vi "Modbusd cmd to db.vi"(0 "reference in":refnum<class "Device.lvclass">, 5 "Data Read":T1, 11 "error in (no error)":errorcluster) -> (4 "reference out":refnum<class "Device.lvclass">, 15 "error out":errorcluster)   [LabVIEW 2019, in "Device.lvclass"]
uses:
  Device.lvclass
  C:/Users/ANENKOV_V1/Desktop/src/Proccess_class/Proccess.lvclass
  Modbus_class/ReadData.ctl
  Proccess_class/Proccess.lvclass/Proccess.ctl
  Logger_class/EventData.ctl
  TypeDef/AlarmType.ctl
  Logger_class/Logger.lvclass
  Proccess_class/Proccess.lvclass
  Modbus_class/ModbusSp.lvclass
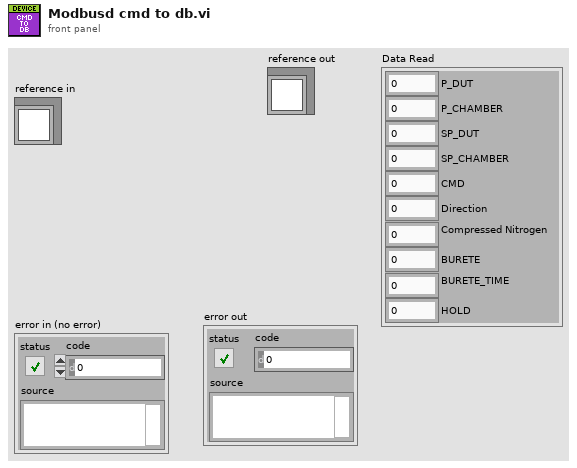
[diagram p1: front panel]
types:
  T1 = typedef "ModbusSp.lvclass/ReadData.ctl" = cluster{"P_DUT":sgl, "P_CHAMBER":sgl, "SP_DUT":sgl, "SP_CHAMBER":sgl, "CMD":u16, "Direction":u16, "Compressed Nitrogen":u16, "BURETE":u16, "BURETE_TIME":u16, "HOLD":u16}
  T2 = typedef "CMD REG.ctl" = cluster{"EXECUTE_SP":bool, "ALARM_PRESS_DOWN_DUT":bool, "ALARM_PRESS_DOWN_CHAMBER":bool, "ALARM_PRESS_DOWN_DUT_CHAMBER":bool, "FILING_DUT":bool, "FILING_CHAMBER":bool, "BLOCK":bool, "PUMP_STATION_OFF":bool, "Leak start":bool, "Leak stop":bool, "Drain":bool}
  T3 = typedef "EventData.ctl" = cluster{"obj_tag":string, "event_tag":string, "Description":string, "ALARM TYPE":T4, "Value DBL":dbl, "Value INT":i32, "Value STR":string, "Time Stamp":timestamp}
  T4 = typedef "AlarmType.ctl" = enum16{"Normal", "Warning", "Alarm"}
  T5 = typedef "Proccess.lvclass/TAGs.ctl" = cluster{"TAG":string, "PTAG":string, "DESC":string}
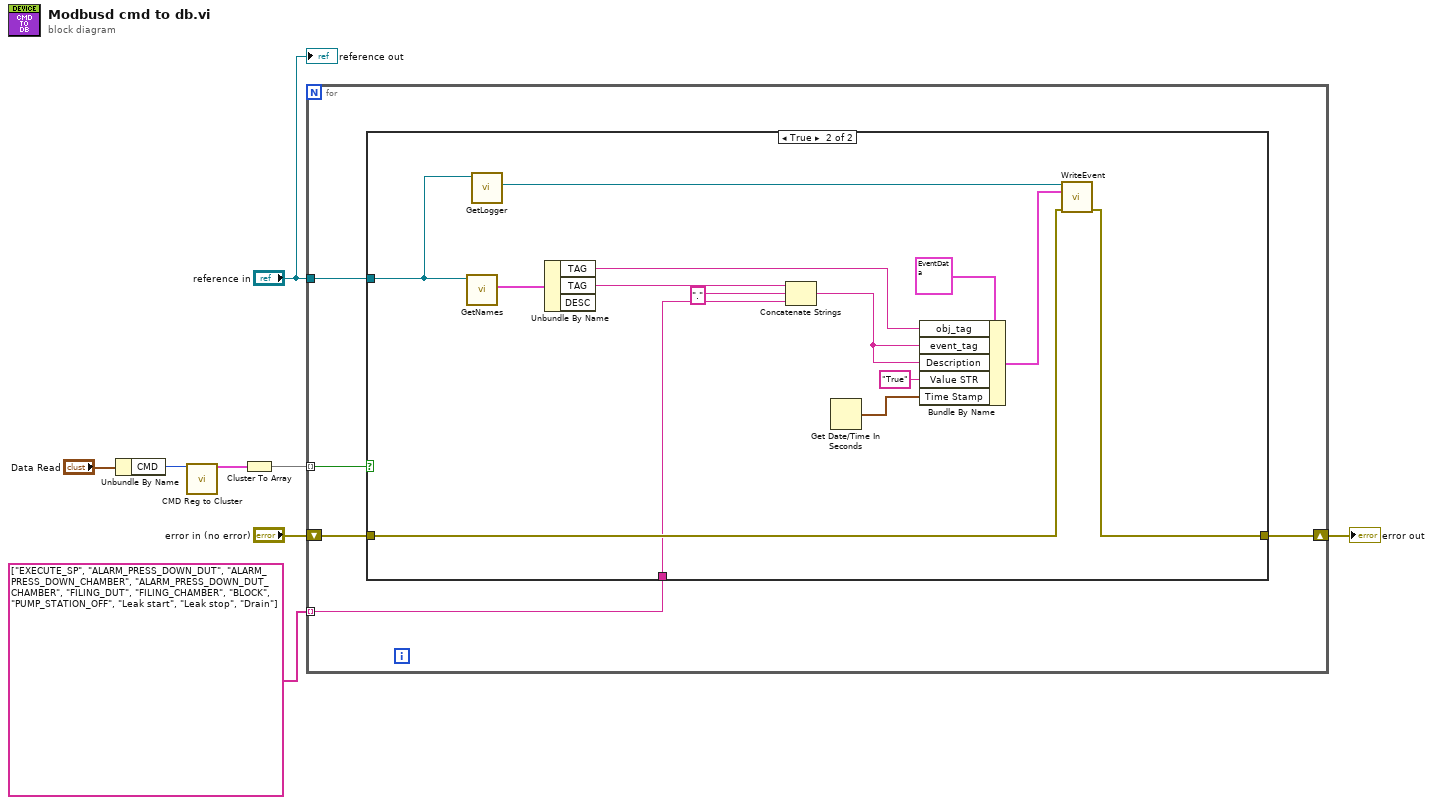
[diagram p0: block diagram]
diagram:
  n1 = Unbundle By Name("Data Read") -> ("CMD"=w4:u16)
  n2 = call "CMD Reg to Cluster.vi"("CMD Reg"=w4) -> ("CMD REG"=w3:T2)  [unwired: 14 in]
  n3 = Cluster To Array(cluster=w3) -> (array=w2:bool[])
  n4 = for {
    tunnel: "reference in" -> [w12]
    shift-right: [w13] -> w8
    shift-left: "error in (no error)" -> [w11]
    tunnel: w2 -> [w10] mode=indexing
    tunnel: string[] ["EXECUTE_SP", "ALARM_PRESS_DOWN_DUT", "ALARM_PRESS_DOWN_CHAMBER", "ALARM_PRESS_DOWN_DUT_CHAMBER", "FILING_DUT", "FILING_CHAMBER", "BLOCK", "PUMP_STATION_OFF", "Leak start", "Leak stop", "Drain"] ("Array") -> [w9] mode=indexing
    n5 = case shown="True" w10 {
      tunnel: [w14 w28] -> w13
      tunnel: w12 -> [_ w27]
      tunnel: w11 -> [w14 w26]
      tunnel: w9 -> [_ w17]
      frame False {
      }
      frame True {
        n6 = call "GetNames.vi"("Proccess in"=w27) -> ("Tags"=w22:T5)  [unwired: 10 in]
        n7 = call "GetLogger.vi"("Proccess in"=w27) -> ("Logger"=w23:refnum<class "Logger.lvclass">)  [unwired: 10 in]
        n8 = Unbundle By Name(w22) -> ("TAG"=w21:string, "TAG"=w20:string)  [unwired: 1 out]
        n9 = Concatenate Strings(w20, "." ("string"), w17) -> (w16:string)
        n10 = Get Date/Time In Seconds() -> (seconds since 1Jan1904=w19:timestamp)
        n11 = Bundle By Name(cluster=T3 {"obj_tag"="", "event_tag"="", "Description"="", "ALARM TYPE"=enum."Normal", "Value DBL"=0.0, "Value INT"=0, "Value STR"="", "Time Stamp"=timestamp(0 s since 1904-01-01)} ("Event"), "obj_tag"=w21, "event_tag"=w16, "Description"=w16, "Value STR"="True", "Time Stamp"=w19) -> (w25:T3)
        n12 = call "WriteEvent.vi"("reference in"=w23, "Event"=w25, "error in (no error)"=w26) -> ("error out"=w28:errorcluster)  [unwired: 11 in, 1 out]
      }
    }
  }
  "error out" <- w8
  "reference out" <- "reference in"
